vi "Correct_Crossconnection_Mistake(111_111)-2.vi"(8 "error IN":errorcluster, 9 "[IN] # of Track with\nFirst Problem Point":i32, 10 "[IN] Index of First Pro\nblem Point Inside Track":i32, 11 "[IN] Still connected\ntracks in group":T2) -> (0 "error OUT":errorcluster, 3 "[OUT] Clusters for Re\nconstructed Tracks":T1, 5 "[OUT] Crossconn\nection corrected":bool)   [LabVIEW 2013]
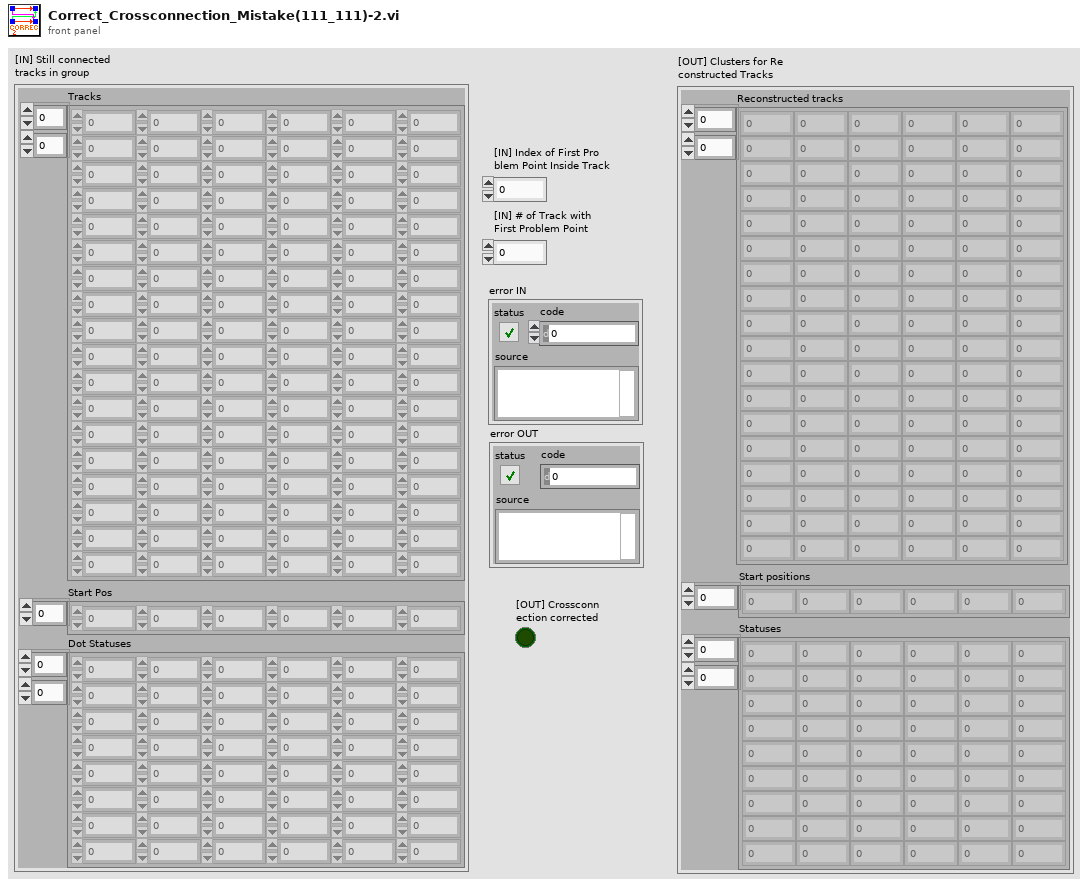
[diagram p1: front panel]
types:
  T1 = cluster{"Reconstructed tracks":dbl[][], "Start positions":i32[], "Statuses":i16[][]}
  T2 = cluster{"Tracks":dbl[][], "Start Pos":i32[], "Dot Statuses":i16[][]}
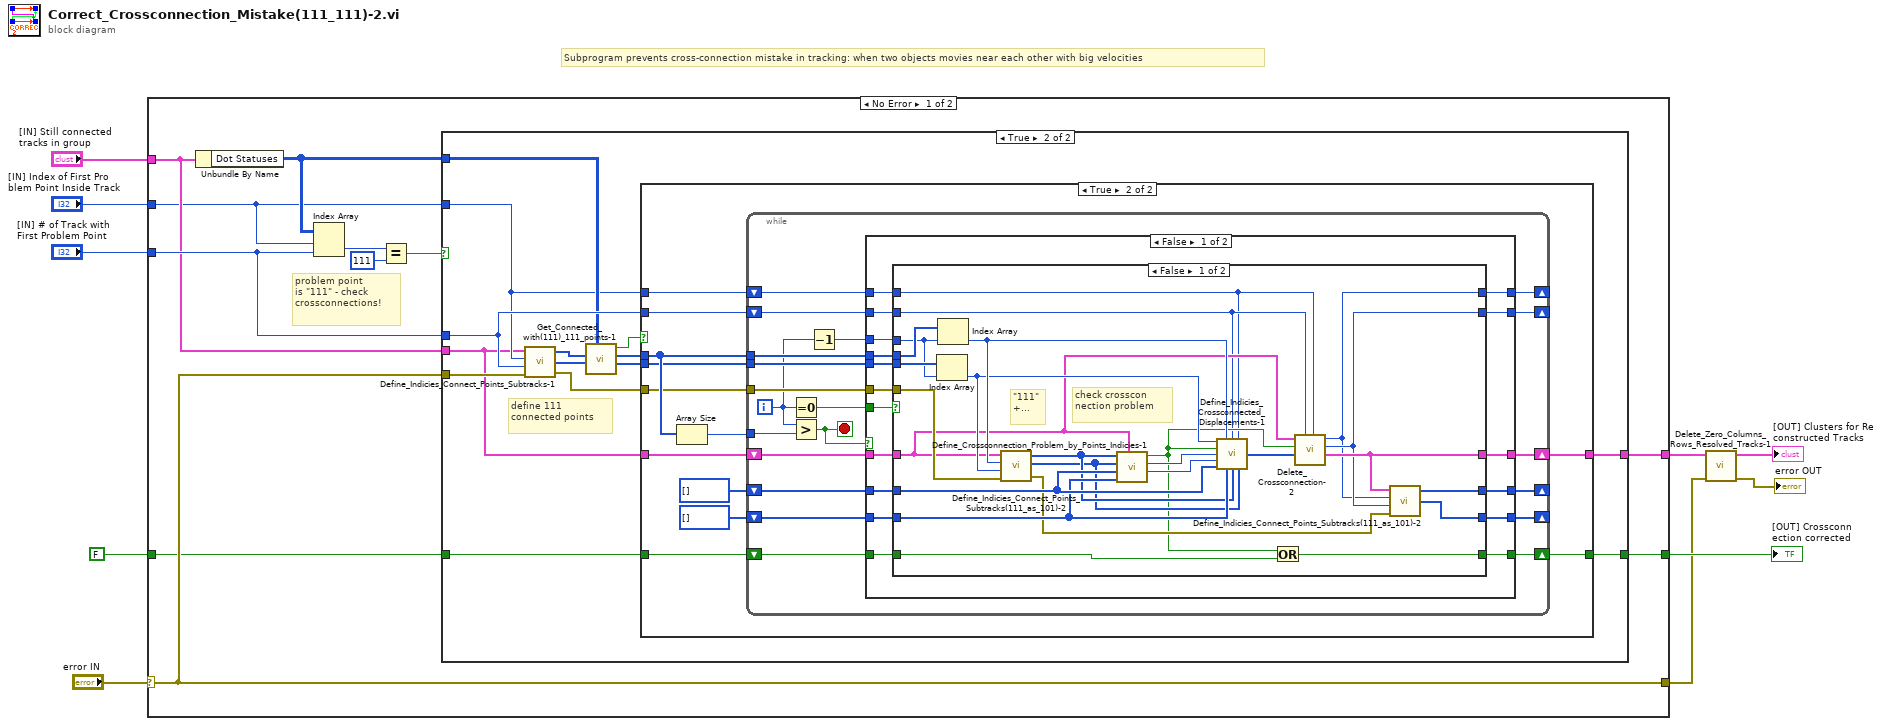
[diagram p0: block diagram]
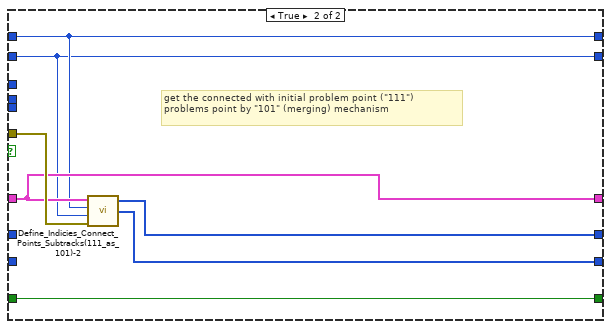
[diagram p4: hidden frame]
diagram:
  # "Subprogram prevents cross-connection mistake in tracking: when two objects movies near each other with big velocities"
  n1 = case shown="No Error" "error IN" {
    selector: "error IN" -> [w20 w129]
    tunnel: [w20 w129] -> w4
    tunnel: [w16 w128] -> w3
    tunnel: "[IN] Index of First Pro\nblem Point Inside Track" -> [w12 _]
    tunnel: "[IN] # of Track with\nFirst Problem Point" -> [w21 _]
    tunnel: FALSE -> [w15 w127]
    tunnel: [w14 w127] -> w6
    tunnel: "[IN] Still connected\ntracks in group" -> [w13 w128]
    frame No Error {
      # "problem point\nis \"111\" - check\ncrossconnections!"
      n2 = Unbundle By Name(w13) -> ("Dot Statuses"=w17:i16[][])
      n3 = Index Array(array=w17, index (row)=w12, index (col)=w21) -> (element=w19:i16)
      n4 = Equal?(x=w19, y=i16 111) -> (x = y?=w11:bool)
      n5 = case shown="True" w11 {
        tunnel: w13 -> [w23 w28]
        tunnel: w20 -> [_ w37]
        tunnel: w12 -> [_ w29]
        tunnel: w21 -> [_ w31]
        tunnel: w17 -> [_ w30]
        tunnel: [w23 w26] -> w16
        tunnel: w15 -> [w22 w25]
        tunnel: [w22 w24] -> w14
        frame False {
        }
        frame True {
          # "define 111\nconnected points"
          n6 = call "Define_Indicies_Connect_Points_Subtracks-1.vi"("error IN"=w37, "[IN] Index of track with\n(problem displacement)"=w31, "[IN] Index of problem\ndisplacement inside track"=w29, "[IN] Track group"=w28) -> ("error OUT"=w27:errorcluster, "[OUT] Index of \nconnected dots\ninside the track"=w35:i32[], "[OUT] Index of connected\ntracks with problem dot"=w36:i32[])
          n7 = call "Get_Connected_with(111)_111_points-1.vi"("[IN] Dot Statuses"=w30, "[IN] Indicies of po\nints inside tracks"=w35, "[IN] Indicies of tracks con\ntaining connected points"=w36) -> ("[OUT] Indicies of tracks co\nntaining connected points"=w32:i32[], "[OUT] Indicies of \npoints inside tracks"=w33:i32[], "[OUT] Candidates for \ncrossconnections are found"=w34:bool)  [unwired: 6 in]
          n8 = case shown="True" w34 {
            tunnel: w33 -> [_ w51]
            tunnel: w32 -> [_ w50]
            tunnel: w31 -> [_ w48]
            tunnel: w29 -> [_ w49]
            tunnel: w28 -> [w39 w47]
            tunnel: w27 -> [_ w46]
            tunnel: [w39 w43] -> w26
            tunnel: w25 -> [w38 w41]
            tunnel: [w38 w40] -> w24
            frame False {
            }
            frame True {
              n9 = Array Size(array=w51) -> (size(s)=w42:i32)
              n10 = while {
                tunnel: w51 -> [w67]
                tunnel: w50 -> [w66]
                tunnel: w46 -> [w60]
                shift-right: [w69] -> _
                shift-left: i32[] [] ("[OUT] Index of connected\ntracks with problem dot") -> [w65]
                shift-right: [w68] -> _
                shift-left: i32[] [] ("[OUT] Index of \nconnected dots\ninside the track") -> [w64]
                shift-right: [w62] -> w43
                shift-left: w47 -> [w63]
                tunnel: w42 -> [w59]
                shift-right: [w55] -> w40
                shift-left: w41 -> [w56]
                shift-right: [w54] -> _
                shift-left: w49 -> [w71]
                shift-right: [w53] -> _
                shift-left: w48 -> [w70]
                i -> [w58]
                stop <- w52 stop-if-true
                n11 = Equal To 0?(x=w58) -> (x = 0?=w61:bool)
                n12 = Greater?(x=w58, y=w59) -> (0:w52:bool)
                n13 = Decrement(x=w58) -> (x-1=w57:i32)
                n14 = case shown="False" w52 {
                  tunnel: w71 -> [w88 w124]
                  tunnel: w70 -> [w87 w123]
                  tunnel: [w86 w126] -> w69
                  tunnel: [w85 w121] -> w68
                  tunnel: w67 -> [w84 _]
                  tunnel: w66 -> [w83 _]
                  tunnel: w65 -> [w82 w126]
                  tunnel: w64 -> [w81 w121]
                  tunnel: w63 -> [w80 w122]
                  tunnel: [w79 w122] -> w62
                  tunnel: w61 -> [w78 _]
                  tunnel: w60 -> [w77 _]
                  tunnel: w57 -> [w76 _]
                  tunnel: w56 -> [w75 w125]
                  tunnel: [w74 w125] -> w55
                  tunnel: [w73 w124] -> w54
                  tunnel: [w72 w123] -> w53
                  frame False {
                    n15 = case shown="False" w78 {
                      tunnel: w88 -> [w89 w115]
                      tunnel: w87 -> [w90 w114]
                      tunnel: w80 -> [w96 w117]
                      tunnel: w77 -> [w113 w120]
                      tunnel: [w98 w119] -> w86
                      tunnel: [w97 w118] -> w85
                      tunnel: w84 -> [w106 _]
                      tunnel: w83 -> [w104 _]
                      tunnel: w82 -> [w110 _]
                      tunnel: w81 -> [w109 _]
                      tunnel: [w93 w117] -> w79
                      tunnel: w76 -> [w103 _]
                      tunnel: w75 -> [w101 w116]
                      tunnel: [w100 w116] -> w74
                      tunnel: [w91 w115] -> w73
                      tunnel: [w92 w114] -> w72
                      frame False {
                        # "\"111\"\n+..."
                        # "check crosscon\nnection problem"
                        n16 = Index Array(array=w104, index=w103) -> (element=w102:i32)
                        n17 = Index Array(array=w106, index=w103) -> (element=w105:i32)
                        n18 = call "Define_Indicies_Connect_Points_Subtracks(111_as_101)-2.vi"("error IN"=w113, "[IN] Index of single track\n(problem displacement)"=w102, "[IN] Index of problem\ndisplacement inside track"=w105, "[IN] Track group"=w96) -> ("error OUT"=w99:errorcluster, "[OUT] Index of \nconnected dots\ninside the track"=w107:i32[], "[OUT] Index of connected\ntracks with problem dot"=w108:i32[])
                        n19 = call "Define_Crossconnection_Problem_by_Points_Indicies-1.vi"("[IN] Track group"=w96, "[IN] Index of connected points \nwith initial point inside the track"=w109, "[IN] Index of connected tra\ncks with initial problem point"=w110, "[IN] Index of connected points \nwith other point inside the track"=w107, "[IN] Index of connected trac\nks with other problem point"=w108) -> ("[OUT] Index in array for \nother problem \"111\" point"=w111:i32, "[OUT] Index in array for \ninitial problem \"111\" point"=w112:i32, "[OUT] The other point \nfor crossconnection found"=w95:bool)  [unwired: 3 in]
                        n20 = call "Define_Indicies_Crossconnected_Displacements-1.vi"("[IN] Index of Track With \nOther Problem Point \"111\""=w102, "[IN] Index of Other Problem \nPoint \"111\" Inside Track"=w105, "[IN] Index of Track with First\n Problem Point"=w90, "[IN] Index of First Pro\nblem Point Inside Track"=w89, "[IN] The other point for\n crossconnection found"=w95, "[IN] Index for initial point"=w112, "[IN] Index for other point"=w111, "[IN] Index of connected tra\ncks with initial problem point"=w110, "[IN] Index of connected points \nwith initial point inside the track"=w109, "[IN] Index of connected trac\nks with other problem point"=w108, "[IN] Index of connected points \nwith other point inside the track"=w107) -> ("[OUT] Indicies of Cross\nconnected Points"=w94:i32[])  [unwired: 4 in]
                        n21 = Or(x=w95, y=w101) -> (x .or. y?=w100:bool)
                        n22 = call "Delete_Crossconnection-2.vi"("[IN] Row index\nInitial Point"=w89, "[IN] Column in\ndex Initial Point"=w90, "[IN] Indicies of Cross\nconnected Points"=w94, "[IN] The other point \nfor crossconnection found"=w95, "[IN] Track group"=w96) -> ("[OUT] Track group"=w93:T2, "[OUT] Column index\nCorrect initial point"=w92:i32, "[OUT] Row index\nCorrect initial point"=w91:i32)  [unwired: 4 in]
                        n23 = call "Define_Indicies_Connect_Points_Subtracks(111_as_101)-2.vi"("error IN"=w99, "[IN] Index of single track\n(problem displacement)"=w92, "[IN] Index of problem\ndisplacement inside track"=w91, "[IN] Track group"=w93) -> ("[OUT] Index of \nconnected dots\ninside the track"=w97:i32[], "[OUT] Index of connected\ntracks with problem dot"=w98:i32[])  [unwired: 1 out]
                      }
                      frame True {
                        # "get the connected with initial problem point (\"111\")\nproblems point by \"101\" (merging) mechanism"
                        n24 = call "Define_Indicies_Connect_Points_Subtracks(111_as_101)-2.vi"("error IN"=w120, "[IN] Index of single track\n(problem displacement)"=w114, "[IN] Index of problem\ndisplacement inside track"=w115, "[IN] Track group"=w117) -> ("[OUT] Index of \nconnected dots\ninside the track"=w118:i32[], "[OUT] Index of connected\ntracks with problem dot"=w119:i32[])  [unwired: 1 out]
                      }
                    }
                  }
                  frame True {
                  }
                }
              }
            }
          }
        }
      }
    }
    frame Error {
    }
  }
  "[OUT] Crossconn\nection corrected" <- w6
  n25 = call "Delete_Zero_Columns_Rows_Resolved_Tracks-1.vi"("error IN"=w4, "[IN] Clusters for Re\nconstructed Tracks"=w3) -> ("error OUT"=→"error OUT":errorcluster, "[OUT] Clusters for Re\nconstructed Tracks"=→"[OUT] Clusters for Re\nconstructed Tracks":T1)  [unwired: 4 in]
